vi "NMEA_ParseMessage-GPGGA.vi"(9 "Error In":errorcluster, 10 "$GPGGA-message_IN":string) -> (1 "Error Out":errorcluster, 2 "$GPGGA-message_OUT":T1={"TimeStamp"=timestamp(0 s since 1904-01-01), "Latitude"=0.0, "Latitude-Direction"=enum."", "Longitude"=1.0, "Longitude-Direction"=enum."", "GPS-Quality"=enum."GPS fix (SPS)", "Number of Satellites"=0, "Horizontal Dilution of Precision"=0.0, "Altitude above Mean-Sea-Level"=0.0, "Geoidal separation"=0.0, "Time since last DGPS update"=0.0, "DGPS reference station ID"=0} {"Time since last DGPS update" format="%.02f [s]"; "Geoidal separation" format="%.02f [m]"; "Altitude above Mean-Sea-Level" format="%.02f [m]"; "Horizontal Dilution of Precision" format="%.02f [HDOP]"; "Longitude" format="%0.4f [long]"; "Latitude" format="%.04f [lat]"; "TimeStamp" format="%<%.2X>T"})   [LabVIEW 2020, in "NMEA.lvlib"]
doc: "<B>GPGGA</B>\nGlobal Positioning System Fix Data"
uses:
  NMEA.lvlib
  NMEA_GPGGA-data.ctl
  NMEA_LatitudeDirection.ctl
  NMEA_LongitudeDirection.ctl
  NMEA_GPS-Quality.ctl
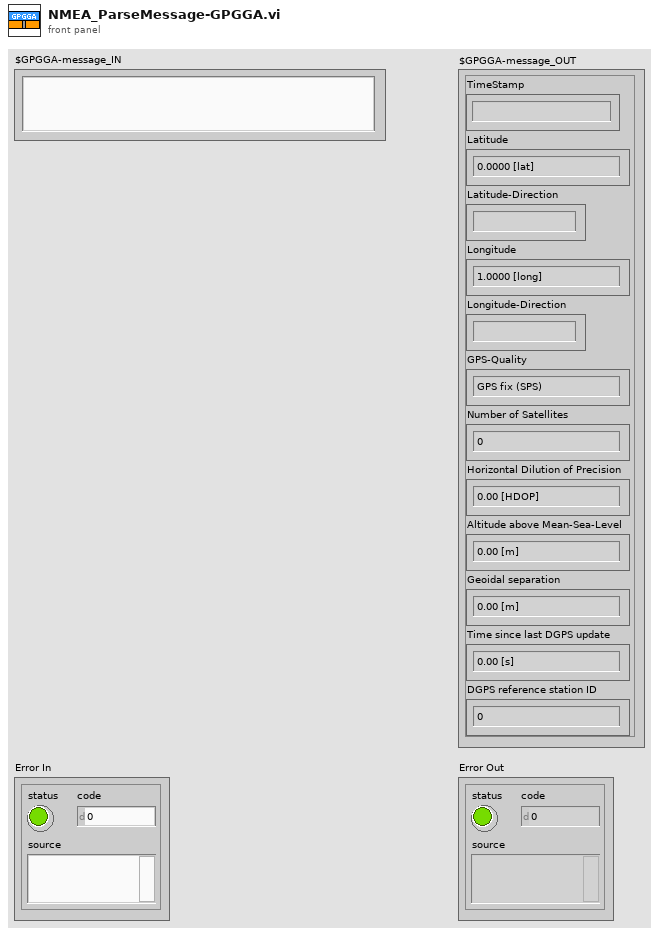
[diagram p1: front panel]
types:
  T1 = typedef "NMEA.lvlib/NMEA_GPGGA-data.ctl" = cluster{"TimeStamp":timestamp, "Latitude":dbl, "Latitude-Direction":T2, "Longitude":dbl, "Longitude-Direction":T3, "GPS-Quality":T4, "Number of Satellites":i32, "Horizontal Dilution of Precision":dbl, "Altitude above Mean-Sea-Level":dbl, "Geoidal separation":dbl, "Time since last DGPS update":dbl, "DGPS reference station ID":i32}
  T2 = typedef "NMEA.lvlib/NMEA_LatitudeDirection.ctl" = enum16{"", "North", "South"}
  T3 = typedef "NMEA.lvlib/NMEA_LongitudeDirection.ctl" = enum16{"", "East", "West"}
  T4 = typedef "NMEA.lvlib/NMEA_GPS-Quality.ctl" = enum16{"Invalid", "GPS fix (SPS)", "DGPS fix", "PPS fix", "Real Time Kinematic", "Float RTK", "estimated", "Manual input mode", "Simulation mode"}
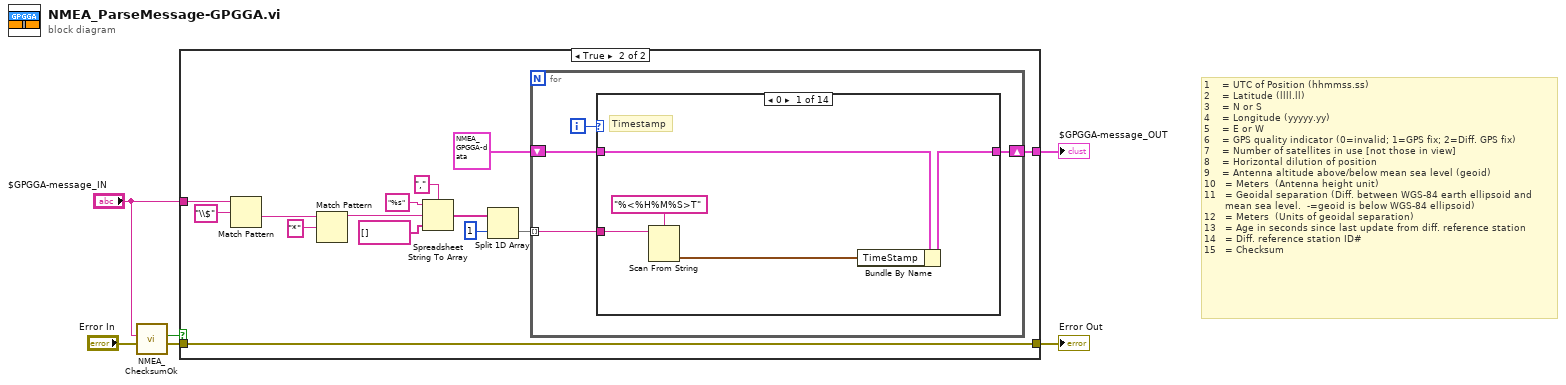
[diagram p0: block diagram]
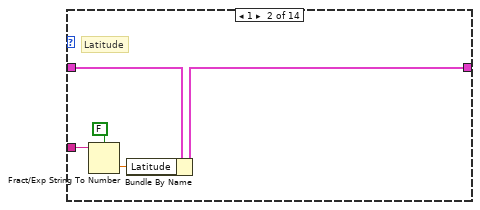
[diagram p3: hidden frame]
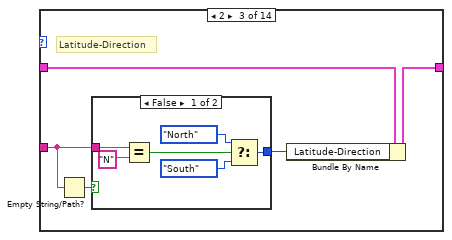
[diagram p4: hidden frame]
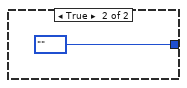
[diagram p5: hidden frame]
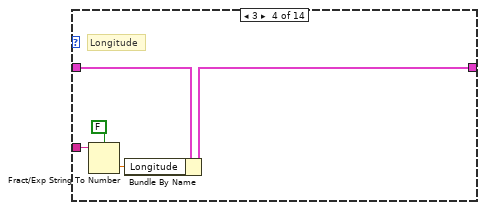
[diagram p6: hidden frame]
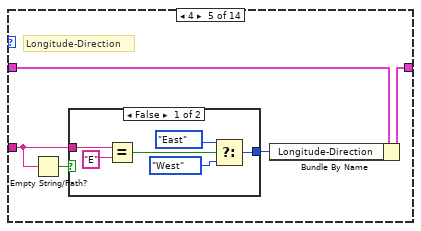
[diagram p7: hidden frame]
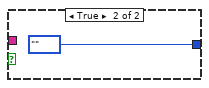
[diagram p8: hidden frame]
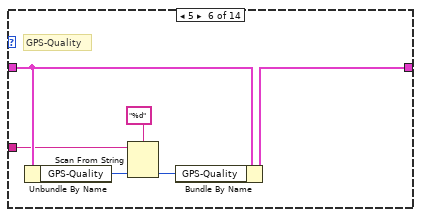
[diagram p9: hidden frame]
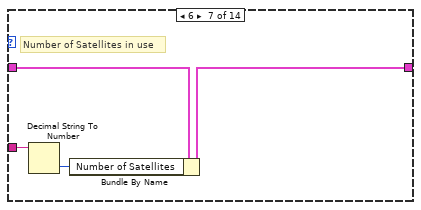
[diagram p10: hidden frame]
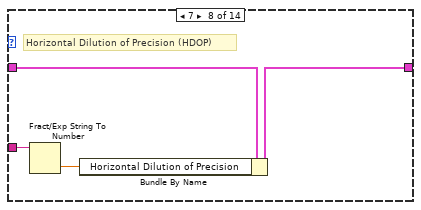
[diagram p11: hidden frame]
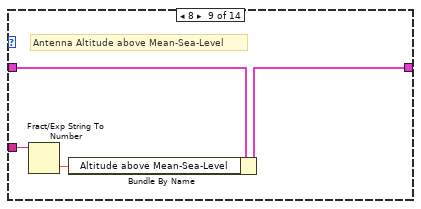
[diagram p12: hidden frame]
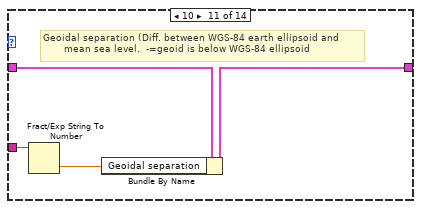
[diagram p14: hidden frame]
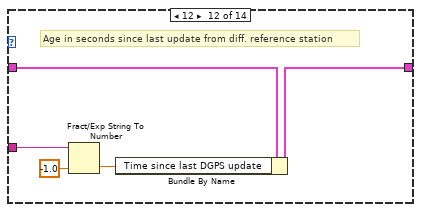
[diagram p15: hidden frame]
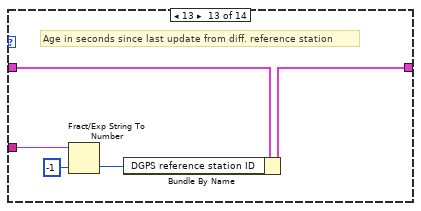
[diagram p16: hidden frame]
diagram:
  # "1    = UTC of Position (hhmmss.ss)\n2    = Latitude (llll.ll)\n3    = N or S\n4    = Longitude (yyyyy.yy)\n5    = E or W\n6    = GPS quality indicator (0=invalid; 1=GPS fix; 2=Diff. GPS fix)\n7    = Number of satellites in use [not those in view]\n8    = Horizontal dilution of position\n9    = Antenna altitude above/below mean sea level (geoid)\n10   = Meters  (Antenna height unit)\n11   = Geoidal separation (Diff. between WGS-84 earth ellipsoid and\n       mean sea level.  -=geoid is below WGS-84 ellipsoid)\n12   = Meters  (Units of geoidal separation)\n13   = Age in seconds since last update from diff. reference station\n14   = Diff. reference station ID#\n15   = Checksum"
  n1 = call "NMEA_ChecksumOk.vi"("Error In"="Error In", "Sentence"="$GPGGA-message_IN") -> ("Error Out"=w1:errorcluster, "CheckSumOk?"=w4:bool)  [unwired: 8 in]
  n2 = case shown="True" w4 {
    tunnel: [_ w16] -> w6
    tunnel: "$GPGGA-message_IN" -> [_ w14]
    tunnel: w1 -> [w7 w9]
    tunnel: [w7 w9] -> w3
    frame False {
    }
    frame True {
      n3 = Match Pattern(string=w14, regular expression="\\$") -> (after substring=w13:string)  [unwired: 1 in, 3 out]
      n4 = Match Pattern(string=w13, regular expression="*") -> (before substring=w20:string)  [unwired: 1 in, 3 out]
      n5 = Spreadsheet String To Array(delimiter (Tab)=",", format string="%s", spreadsheet string=w20, array type (2D Dbl)=string[] []) -> (array=w11:string[])
      n6 = Split 1D Array(array=w11, index=1) -> (second subarray=w12:string[])  [unwired: 1 out]
      n7 = for {
        tunnel: w12 -> [w22] mode=indexing
        shift-right: [w24] -> w16
        shift-left: T1 {"TimeStamp"=timestamp(0 s since 1904-01-01), "Latitude"=0.0, "Latitude-Direction"=enum."", "Longitude"=1.0, "Longitude-Direction"=enum."", "GPS-Quality"=enum."GPS fix (SPS)", "Number of Satellites"=0, "Horizontal Dilution of Precision"=0.0, "Altitude above Mean-Sea-Level"=0.0, "Geoidal separation"=0.0, "Time since last DGPS update"=0.0, "DGPS reference station ID"=0} ("$GPGGA-message_OUT") -> [w25]
        i -> [w23]
        n8 = case shown="0" w23 {
          tunnel: w25 -> [w30 w35 w40 w52 w57 w69 w74 w78 w82 w83 w87 w92 w97 w98]
          tunnel: [w29 w34 w39 w51 w56 w70 w73 w77 w81 w83 w86 w91 w96 w98] -> w24
          tunnel: w22 -> [w27 w33 w37 w50 w54 w66 w72 w76 w80 _ w85 w90 w95 _]
          frame 0 {
            # "Timestamp"
            n9 = Scan From String(format string="%<%H%M%S>T", input string=w27) -> (output 1=w26:timestamp)  [unwired: 3 in, 3 out]
            n10 = Bundle By Name(cluster=w30, "TimeStamp"=w26) -> (w29:T1)
          }
          frame 1 {
            # "Latitude"
            n11 = Fract/Exp String To Number(use system decimal point (T)=FALSE, string=w33) -> (number=w32:dbl)  [unwired: 2 in, 1 out]
            n12 = Bundle By Name(cluster=w35, "Latitude"=w32) -> (w34:T1)
          }
          frame 2 {
            # "Latitude-Direction"
            n13 = Empty String/Path?(string/path=w37) -> (empty?=w36:bool)
            n14 = case shown="False" w36 {
              tunnel: [w43 NMEA_LatitudeDirection."" ("f")] -> w38
              tunnel: w37 -> [w41 _]
              frame False {
                n15 = Equal?(x=w41, y="N") -> (x = y?=w45:bool)
                n16 = Select(t=NMEA_LatitudeDirection."North" ("Latitude-Direction"), s=w45, f=NMEA_LatitudeDirection."South") -> (s? t:f=w43:T2)
              }
              frame True {
              }
            }
            n17 = Bundle By Name(cluster=w40, "Latitude-Direction"=w38) -> (w39:T1)
          }
          frame 3 {
            # "Longitude"
            n18 = Fract/Exp String To Number(use system decimal point (T)=FALSE, string=w50) -> (number=w49:dbl)  [unwired: 2 in, 1 out]
            n19 = Bundle By Name(cluster=w52, "Longitude"=w49) -> (w51:T1)
          }
          frame 4 {
            # "Longitude-Direction"
            n20 = Empty String/Path?(string/path=w54) -> (empty?=w53:bool)
            n21 = case shown="False" w53 {
              tunnel: w54 -> [w63 _]
              tunnel: [w59 NMEA_LongitudeDirection."" ("f")] -> w55
              frame False {
                n22 = Equal?(x=w63, y="E") -> (x = y?=w61:bool)
                n23 = Select(t=NMEA_LongitudeDirection."East" ("Longitude-Direction"), s=w61, f=NMEA_LongitudeDirection."West") -> (s? t:f=w59:T3)
              }
              frame True {
              }
            }
            n24 = Bundle By Name(cluster=w57, "Longitude-Direction"=w55) -> (w56:T1)
          }
          frame 5 {
            # "GPS-Quality"
            n25 = Unbundle By Name(w69) -> ("GPS-Quality"=w68:T4)
            n26 = Scan From String(format string="%d", input string=w66, default 1=w68) -> (output 1=w67:T4)  [unwired: 2 in, 3 out]
            n27 = Bundle By Name(cluster=w69, "GPS-Quality"=w67) -> (w70:T1)
          }
          frame 6 {
            # "Number of Satellites in use"
            n28 = Decimal String To Number(string=w72) -> (number=w71:i32)  [unwired: 2 in, 1 out]
            n29 = Bundle By Name(cluster=w74, "Number of Satellites"=w71) -> (w73:T1)
          }
          frame 7 {
            # "Horizontal Dilution of Precision (HDOP)"
            n30 = Fract/Exp String To Number(string=w76) -> (number=w75:dbl)  [unwired: 3 in, 1 out]
            n31 = Bundle By Name(cluster=w78, "Horizontal Dilution of Precision"=w75) -> (w77:T1)
          }
          frame 8 {
            # "Antenna Altitude above Mean-Sea-Level"
            n32 = Fract/Exp String To Number(string=w80) -> (number=w79:dbl)  [unwired: 3 in, 1 out]
            n33 = Bundle By Name(cluster=w82, "Altitude above Mean-Sea-Level"=w79) -> (w81:T1)
          }
          frame 9, 11 {
            # "[9] - Meters (antenna height unit)\n[11] - Meters (units of geoidal separation)"
          }
          frame 10 {
            # "Geoidal separation (Diff. between WGS-84 earth ellipsoid and\n       mean sea level.  -=geoid is below WGS-84 ellipsoid"
            n34 = Fract/Exp String To Number(string=w85) -> (number=w84:dbl)  [unwired: 3 in, 1 out]
            n35 = Bundle By Name(cluster=w87, "Geoidal separation"=w84) -> (w86:T1)
          }
          frame 12 {
            # "Age in seconds since last update from diff. reference station"
            n36 = Fract/Exp String To Number(string=w90, default (0 dbl)=-1.0 ("default (0 DBL)")) -> (number=w89:dbl)  [unwired: 2 in, 1 out]
            n37 = Bundle By Name(cluster=w92, "Time since last DGPS update"=w89) -> (w91:T1)
          }
          frame 13 {
            # "Age in seconds since last update from diff. reference station"
            n38 = Fract/Exp String To Number(string=w95, default (0 dbl)=-1 ("DGPS reference station ID")) -> (number=w94:i32)  [unwired: 2 in, 1 out]
            n39 = Bundle By Name(cluster=w97, "DGPS reference station ID"=w94) -> (w96:T1)
          }
          frame Default {
          }
        }
      }
    }
  }
  "$GPGGA-message_OUT" <- w6
  "Error Out" <- w3
